vi "Single Engine Main.vi"() -> ()   [LabVIEW 2013]
uses:
  <vilib>/NI/Module Execution Interface/Engine Runtime/Execution States.ctl
  <vilib>/NI/Module Execution Interface/Engine Runtime/Engine Runtime Interface.lvclass
  <vilib>/NI/Tag Bus Data Framework/Framework Configuration Classes/target runtime/PL_Target Runtime.lvclass
  <vilib>/rvi/interface/nirviOpenFPGA/nirviOpenFPGA.xnode
  <vilib>/NI/Tag Bus Module Framework/FPGA manager/FPGA manager.lvlib
  <vilib>/NI/Tag Bus Module Framework/FPGA manager/methods.ctl
  <vilib>/userdefined/High Color/nirio_resource_hc.ctl
  <vilib>/NI/Configuration Framework/tree serializer/NISE_CEF_TreeSerializer.lvlib
  <vilib>/NI/Tag Bus Data Framework/Framework Configuration Classes/flattened data interface/PL_Serialization Interface.lvlib
panel:
  in  "target":i32
  out "final error":errorcluster
  in  "stop":bool
  out "runtime error":errorcluster
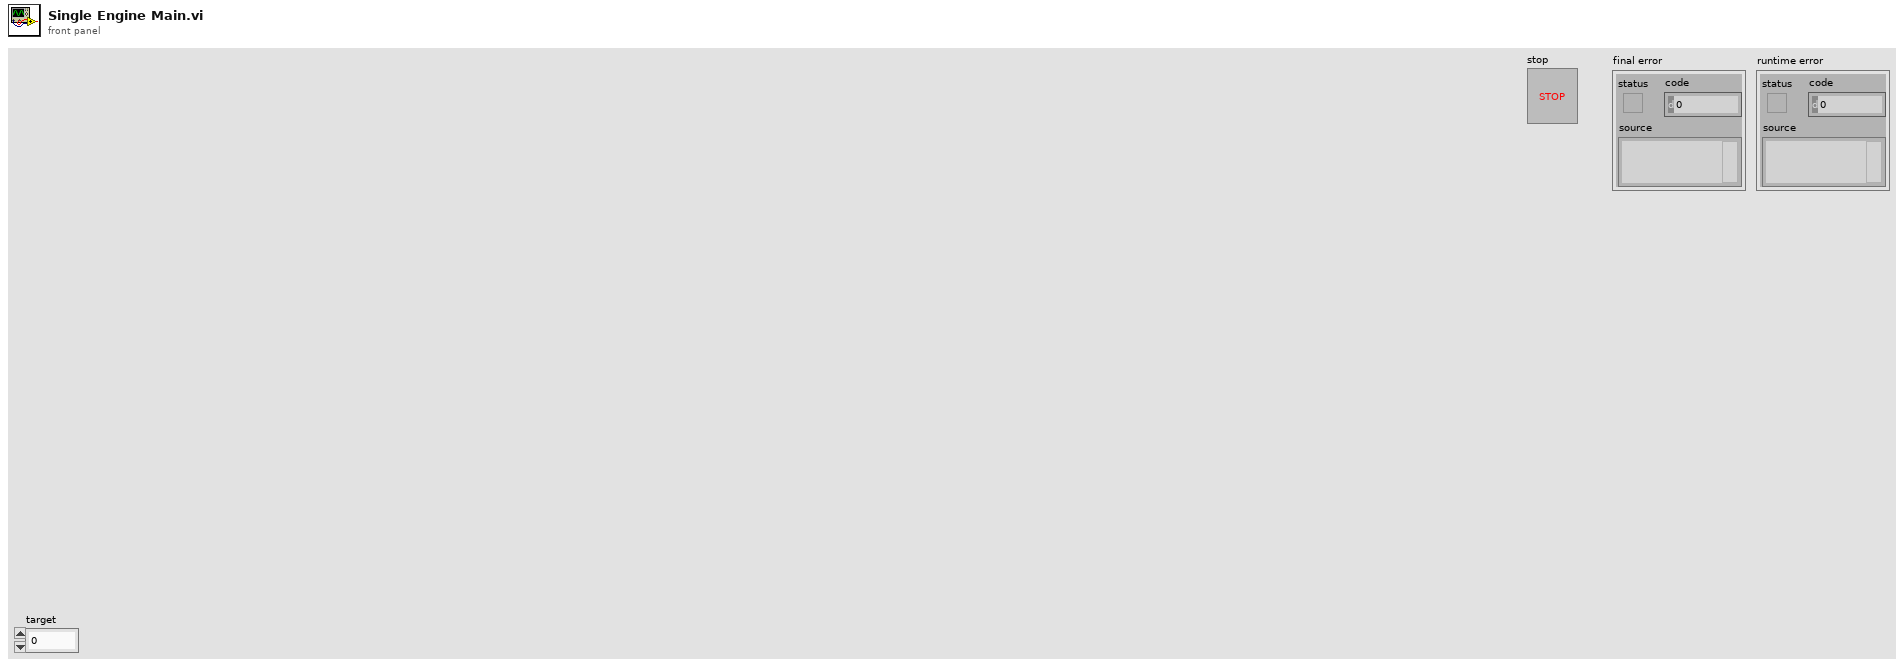
[diagram p1: front panel]
types:
  T1 = typedef "nirio_resource_hc.ctl" = tag
  T2 = typedef "FPGA manager.lvlib/methods.ctl" = enum16{"initialize bitfile", "cache bitfile", "locate bitfile", "close bitfile"}
  T3 = typedef "NISE_CEF_TreeSerializer.lvlib/base file format.ctl" = cluster{"version":string, "data":string}
  T4 = typedef "NISE_CEF_TreeSerializer.lvlib/flat hierarchy.ctl" = cluster{"hierarchy structure":T5, "instance data":T7[]}
  T5 = typedef "NISE_CEF_TreeSerializer.lvlib/full hierarchy.ctl" = cluster{"root":string, "hierarchy":T6[]}
  T6 = typedef "NISE_CEF_TreeSerializer.lvlib/hierarchy element.ctl" = cluster{"current node":string, "children":string[]}
  T7 = typedef "NISE_CEF_TreeSerializer.lvlib/instance data.ctl" = cluster{"ID":string, "Alias":string, "class":string, "version":string, "data":string}
  T8 = typedef "PLConfigurationSerializer.lvlib/targets cluster.ctl" = cluster{"Target Configuration":refnum<class "PL_Target Configuration.lvclass">, "engines":T9[]}
  T9 = typedef "PLConfigurationSerializer.lvlib/engines cluster.ctl" = cluster{"engine configuration":refnum<class "engine configuration.lvclass">, "modules":refnum<class "TBM module configuration.lvclass">[]}
  T10 = typedef "Engine Runtime Interface.lvclass/Execution States.ctl" = enum16{"Initializing", "Paused (Initialized)", "Running", "Set Safe Outputs", "Uninitializing", "Stopped (Uninitialized)", "Error (Uninitialized)", "Safe State (Uninitialized)", "Closed"}
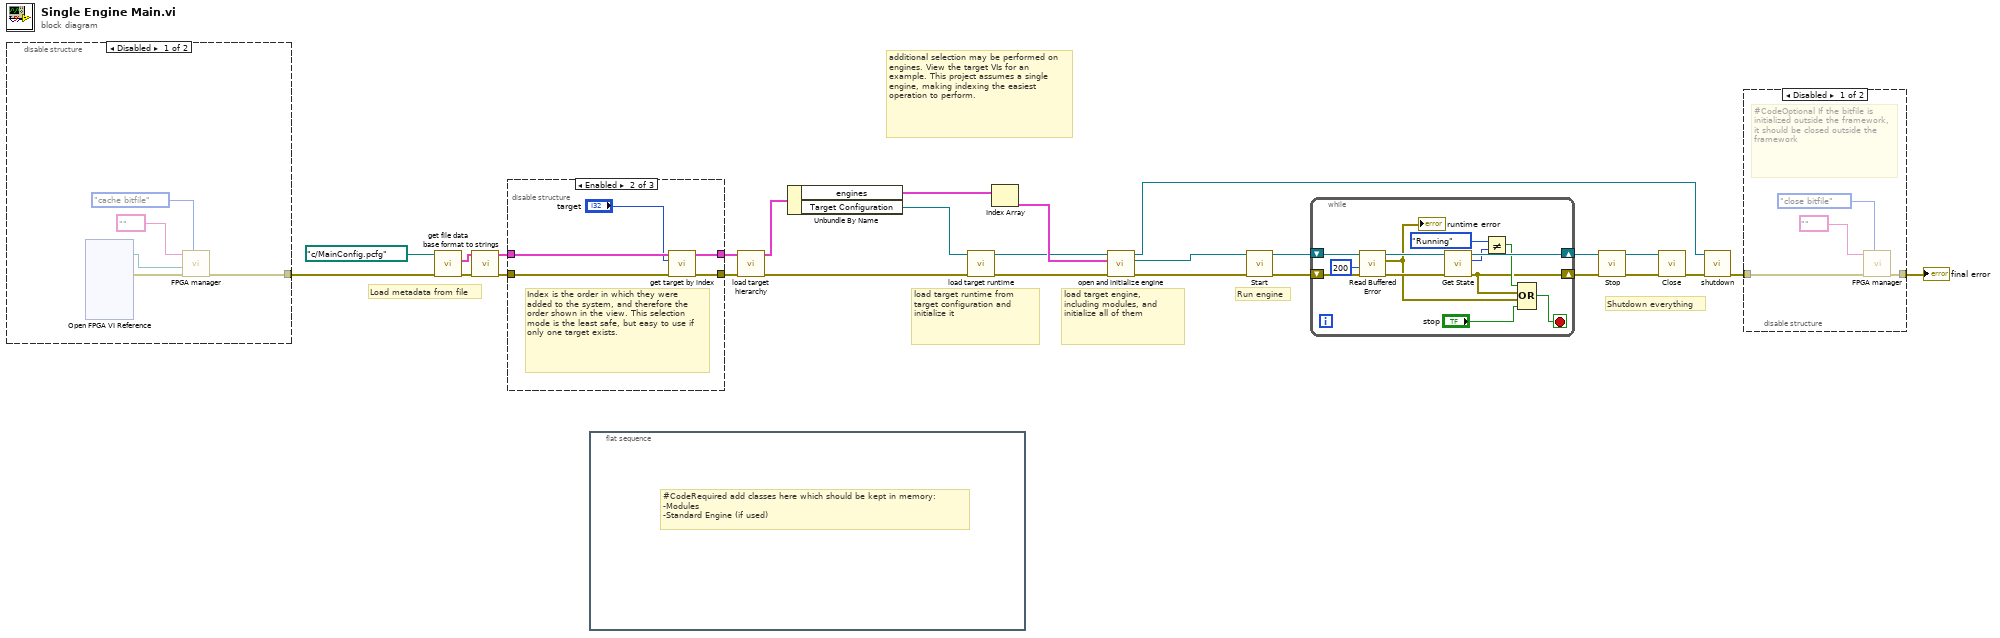
[diagram p0: block diagram]
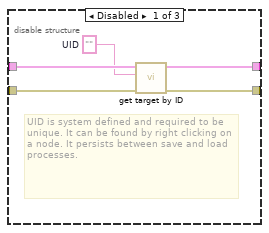
[diagram p2: hidden frame]
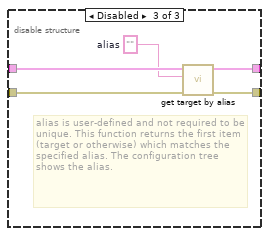
[diagram p3: hidden frame]
diagram:
  # "additional selection may be performed on engines. View the target VIs for an example. This project assumes a single engine, making indexing the easiest operation to perform."
  # "Shutdown everything"
  # "Run engine"
  # "load target engine, including modules, and initialize all of them"
  # "load target runtime from target configuration and initialize it"
  # "Load metadata from file"
  n1 = disable-structure shown="Disabled" {
    disable-tunnel: [w28 _] -> w8
    frame Disabled {
      n2 = xnode "Open FPGA VI Reference"() -> ("FPGA VI Reference Out"=w31:refnum<k20>, "error out"=w32:errorcluster)  [unwired: 2 in]
      n3 = call <vilib>:"FPGA manager.vi"("action"=methods."cache bitfile", "error in"=w32, "bitfile to cache"=w31, "RIO resource"=T1 "") -> ("error out"=w28:errorcluster)  [unwired: 5 in, 2 out]
    }
    frame Enabled {
    }
  }
  n4 = call <vilib>:"get file data.vi"("error in"=w8, "Path"=path "c:/MainConfig.pcfg" ("file path")) -> ("error out"=w10:errorcluster, "format"=w9:T3)  [unwired: 8 in]
  n5 = call <vilib>:"base format to strings.vi"("error in"=w10, "format"=w9) -> ("error out"=w6:errorcluster, "data"=w5:T4)  [unwired: 8 in]
  n6 = disable-structure shown="Enabled" {
    disable-tunnel: w6 -> [w36 w39 w44]
    disable-tunnel: w5 -> [w37 w40 w45]
    disable-tunnel: [w34 w42 w47] -> w4
    disable-tunnel: [w33 w41 w46] -> w3
    frame Disabled {
      w35 = ""  # UID
      # "UID is system defined and required to be unique. It can be found by right clicking on a node. It persists between save and load processes."
      n7 = call <vilib>:"get target by ID.vi"("error in"=w36, "UID"=w35, "full system"=w37) -> ("error out"=w33:errorcluster, "target hierarchy"=w34:T4)  [unwired: 7 in]
    }
    frame Enabled {
      # "Index is the order in which they were added to the system, and therefore the order shown in the view. This selection mode is the least safe, but easy to use if only one target exists."
      n8 = call <vilib>:"get target by index.vi"("error in"=w39, "index"="target", "system hierarchy"=w40) -> ("error out"=w41:errorcluster, "target hierarchy"=w42:T4)  [unwired: 7 in]
    }
    frame Disabled {
      w43 = ""  # alias
      # "alias is user-defined and not required to be unique. This function returns the first item (target or otherwise) which matches the specified alias. The configuration tree shows the alias."
      n9 = call <vilib>:"get target by alias.vi"("error in"=w44, "alias"=w43, "system hierarchy"=w45) -> ("error out"=w46:errorcluster, "target hierarchy"=w47:T4)  [unwired: 7 in]
    }
  }
  n10 = flat-sequence {
    frame #0 {
      # "#CodeRequired add classes here which should be kept in memory:\n-Modules\n-Standard Engine (if used)"
      # "Add classes here to be in memory"
    }
  }
  n11 = call <vilib>:"load target hierarchy.vi"("error in"=w3, "target hierarchy"=w4) -> ("error out"=w2:errorcluster, "targets cluster out"=w1:T8)  [unwired: 8 in]
  n12 = Unbundle By Name(w1) -> ("engines"=w21:T9[], "Target Configuration"=w15:refnum<class "PL_Target Configuration.lvclass">)
  n13 = call <vilib>:"load target runtime.vi"("error in"=w2, "target configuration"=w15) -> ("error out"=w14:errorcluster, "target runtime"=w13:refnum<class "PL_Target Runtime.lvclass">)  [unwired: 8 in]
  n14 = Index Array(array=w21) -> (element=w16:T9)  [unwired: 1 in]
  n15 = call <vilib>:"open and initialize engine.vi"("error in"=w14, "engine configuration in"=w16, "Target Runtime in"=w13) -> ("error out"=w20:errorcluster, "Engine Runtime Interface out"=w19:refnum<class "Engine Runtime Interface.lvclass">, "Target Runtime out"=w17:refnum<class "PL_Target Runtime.lvclass">)  [unwired: 6 in]
  n16 = call-dynamic "Start.vi"("error in"=w20, "Engine Runtime Interface in"=w19) -> ("error out"=w22:errorcluster, "Engine Runtime Interface out"=w25:refnum<class "Engine Runtime Interface.lvclass">)  [unwired: 8 in]
  n17 = while {
    shift-right: [w56] -> w24
    shift-left: w25 -> [w60]
    shift-right: [w49] -> w23
    shift-left: w22 -> [w59]
    stop <- w54 stop-if-true
    n18 = call-dynamic "Read Buffered Error.vi"("error in"=w59, "timeout in ms (0)"=200, "Engine Runtime Interface in"=w60) -> ("error out"=w57:errorcluster, "Engine Error"=w53:errorcluster, "Engine Runtime Interface out"=w58:refnum<class "Engine Runtime Interface.lvclass">)  [unwired: 6 in]
    "runtime error" <- w53
    n19 = call-dynamic "Get State.vi"("error in"=w57, "Engine Runtime Interface in"=w58) -> ("error out"=w49:errorcluster, "Engine State"=w52:T10, "Engine Runtime Interface out"=w56:refnum<class "Engine Runtime Interface.lvclass">)  [unwired: 7 in]
    n20 = Not Equal?(x=Execution_States."Running" ("Engine State"), y=w52) -> (x != y?=w50:bool)
    n21 = Compound Arithmetic op=OR(w50, w49, w53, "stop") -> (w54:bool)
  }
  n22 = call-dynamic "Stop.vi"("error in"=w23, "Engine Runtime Interface in"=w24) -> ("error out"=w26:errorcluster, "Engine Runtime Interface out"=w27:refnum<class "Engine Runtime Interface.lvclass">)  [unwired: 8 in]
  n23 = call-dynamic "Close.vi"("error in"=w26, "Engine Runtime Interface in"=w27) -> ("error out"=w18:errorcluster)  [unwired: 9 in]
  n24 = call-dynamic "shutdown.vi"("error in"=w18, "Target Runtime in"=w17) -> ("error out"=w12:errorcluster)  [unwired: 9 in]
  n25 = disable-structure shown="Disabled" {
    disable-tunnel: w12 -> [w62 w65]
    disable-tunnel: [w61 w65] -> w11
    frame Disabled {
      # "#CodeOptional If the bitfile is initialized outside the framework, it should be closed outside the framework"
      n26 = call <vilib>:"FPGA manager.vi"("action"=methods."close bitfile", "error in"=w62, "RIO resource"=T1 "") -> ("error out"=w61:errorcluster)  [unwired: 6 in, 2 out]
    }
    frame Enabled {
    }
  }
  "final error" <- w11
